vi "Contour Defect Inspection.vi"() -> ()   [LabVIEW 2016]
doc: "This example shows a contour analysis application. The contour of the rim of the can is extracted and a circle is fitted to those points. Then the contour is compared to the fitted circle to locate defects."
uses:
  <vilib>/vision/NI_Vision_Development_Module.lvlib
panel:
  out "Pass Status":bool
  in  "Max Distance":dbl=4.0 min=0.0 format="%.2f"
  out "Distance":dbl[](graph) caption="Distance of Contour from Fitted Circle"
  in  "Stop":bool
  out "Image":T1(plugin-control)
  in  "Delay (s.)":dbl(slide)=0.995260663507109 scale=0.0..3.0
  # "Overview: Demonstrates how to use the IMAQ Fit Contour function to compare the extracted contour against an expected shape contour and IMAQ Compute Contour Distance calculates the distance of the contour points from the expected shape.\nRequirements: Vision Development Software.\nInstructions:\n1. Run the VI.\n2. Adjust the Max Distance to change the distance tolerance. The locations that are greater than this maximum distance are overlaid in red on the image."
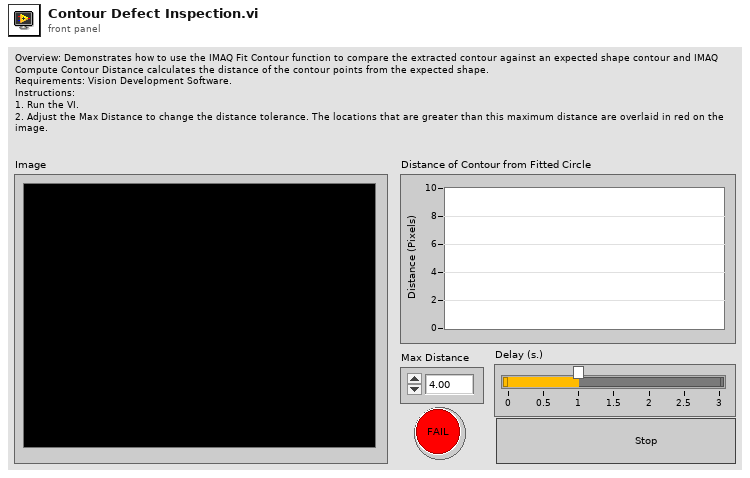
[diagram p1: front panel]
types:
  T1 = typedef "IMAQ Image.ctl" = refnum<image>
  T2 = typedef "IMAQ Circle" = cluster{"Center X":i32, "Center Y":i32, "Inner Radius":i32, "Outer Radius":i32, "Start Angle":dbl, "End Angle":dbl}
  T3 = typedef "ROI Descriptor" = cluster{"Global Rectangle":i32[], "Contours":cluster{"ID":enum32{"External", "Internal"}, "Type":u32, "Coordinates":i32[]}[]}
  T4 = cluster{"Overlay?":bool, "Color":u32, "Width":u32, "Maintain Width?":bool}
  T5 = enum16{"Closest To Search Start", "Maximum Length", "Strongest Mean Gradient Change"}
  T6 = enum16{"Rect Left To Right", "Rect Right To Left", "Rect Top To Bottom", "Rect Bottom To Top", "Annulus Inner To Outer", "Annulus Outer To Inner", "Annulus Start Angle To End Angle", "Annulus End Angle To Start Angle"}
  T7 = cluster{"Target Point":cluster{"X":dbl, "Y":dbl}, "Template Point":cluster{"X":dbl, "Y":dbl}, "Distance":dbl}[]
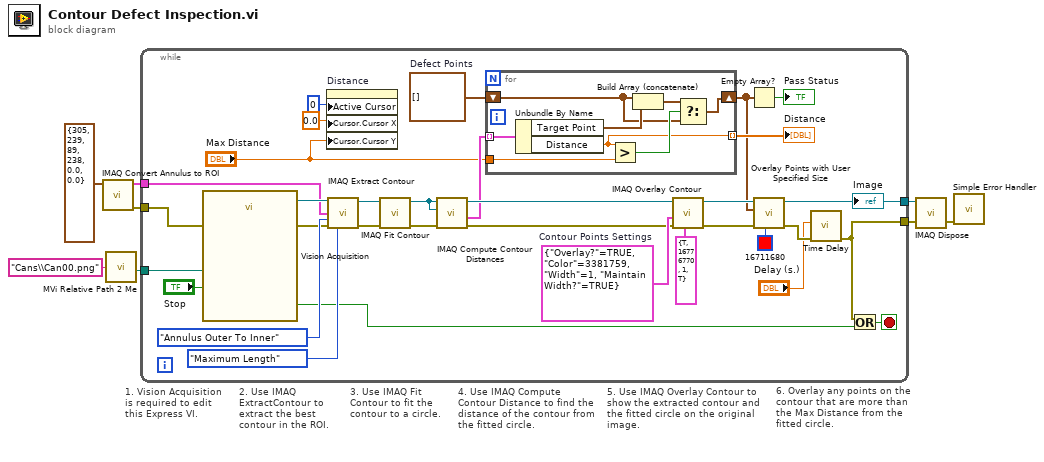
[diagram p0: block diagram]
diagram:
  # "1. Vision Acquisition is required to edit this Express VI."
  # "6. Overlay any points on the contour that are more than the Max Distance from the fitted circle."
  # "4. Use IMAQ Compute Contour Distance to find the distance of the contour from the fitted circle."
  # "3. Use IMAQ Fit Contour to fit the contour to a circle."
  # "5. Use IMAQ Overlay Contour to show the extracted contour and the fitted circle on the original image."
  # "2. Use IMAQ ExtractContour to extract the best contour in the ROI."
  n1 = call "IMAQ Convert Annulus to ROI"("Annulus"=T2 {"Center X"=305, "Center Y"=239, "Inner Radius"=89, "Outer Radius"=238, "Start Angle"=0.0, "End Angle"=0.0}) -> ("error out"=w3:errorcluster, "ROI Descriptor"=w6:T3)  [unwired: 8 in]
  n2 = call "MVi Relative Path 2 Me.vi"("Relative Path"="Cans\\Can00.png" ("name or relative path")) -> ("Appended Dir"=w2:path)  [unwired: 5 in, 1 out]
  n3 = while {
    tunnel: [w25] -> w8
    tunnel: w2 -> [w22]
    tunnel: w6 -> [w21]
    tunnel: [w11] -> w5
    tunnel: w3 -> [w12]
    stop <- w10 stop-if-true
    w28 = cluster{"X":dbl, "Y":dbl}[] []  # Defect Points
    w38 = T4 {"Overlay?"=TRUE, "Color"=3381759, "Width"=1, "Maintain Width?"=TRUE}  # Contour Points Settings
    n4 = call "Vision Acquisition"("Image Path"=w22, "Stop (F)"="Stop", "error in"=w12) -> ("Image Out"=w24:T1, "Stopped"=w9:bool, "error out"=w23:errorcluster)  [unwired: 22 in]
    n5 = property on="Distance" class="WFGraph (strict)"("Active Cursor"=u32 0, "Cursor.Cursor X"=0.0 ("Cursor.Cursor Position:Cursor X"), "Cursor.Cursor Y"="Max Distance") -> ()  [unwired: 2 in, 2 out]
    n6 = call "IMAQ Extract Contour"("Source Image"=w24, "ROI Descriptor"=w21, "Search Direction"=T6."Annulus Outer To Inner", "error in (no error)"=w23, "Contour Selection"=T5."Maximum Length") -> ("Source Image Out"=w34:T1, "error out"=w33:errorcluster)  [unwired: 3 in, 6 out]
    n7 = call-poly "IMAQ Fit Contour"("error in (no error)"=w33, "Contour Image"=w34) -> ("error out"=w39:errorcluster, "Contour Image Out"=w30:T1)  [unwired: 2 in, 6 out]
    n8 = call "IMAQ Compute Contour Distances"("error in (no error)"=w39, "Template Contour Image"=w30, "Target Contour Image"=w30) -> ("error out"=w35:errorcluster, "Distances"=w29:T7, "Target Contour Image Out (dup)"=w36:T1)  [unwired: 2 in, 4 out]
    n9 = for {
      tunnel: w29 -> [w49] mode=indexing
      shift-right: [w44] -> w19
      shift-left: w28 -> [w45]
      tunnel: [w43] -> w20 mode=indexing
      tunnel: "Max Distance" -> [w42]
      n10 = Unbundle By Name(w49) -> ("Target Point"=w48:cluster{"X":dbl, "Y":dbl}, "Distance"=w43:dbl)
      n11 = Greater?(x=w43, y=w42) -> (0:w47:bool)
      n12 = Build Array (concatenate)(w45, w48) -> (w46:cluster{"X":dbl, "Y":dbl}[])
      n13 = Select(t=w46, s=w47, f=w45) -> (s? t:f=w44:cluster{"X":dbl, "Y":dbl}[])
    }
    "Distance" <- w20
    n14 = call "IMAQ Overlay Contour"("Contour Equation Settings"=T4 {"Overlay?"=TRUE, "Color"=16776770, "Width"=1, "Maintain Width?"=TRUE}, "error in (no error)"=w35, "Contour Points Settings"=w38, "Image"=w36) -> ("error out"=w13:errorcluster, "Image Out"=w27:T1)  [unwired: 2 in, 4 out]
    n15 = Empty Array?(array=w19) -> (empty?=→"Pass Status":bool)
    n16 = call "Overlay Points with User Specified Size.vi"("Color"=u32 16711680, "error in"=w13, "Points"=w19, "Image In"=w27) -> ("error out"=w15:errorcluster, "Image Out"=w25:T1)  [unwired: 6 in]
    "Image" <- w25
    n17 = call "Time Delay"("error in (no error)"=w15, "Delay Time (s)"="Delay (s.)") -> ("error out"=w11:errorcluster)  [unwired: 9 in]
    n18 = Or(x=w11, y=w9) -> (x .or. y?=w10:bool)
  }
  n19 = call "IMAQ Dispose"("Image"=w8, "error in (no error)"=w5) -> ("error out"=w4:errorcluster)  [unwired: 1 in, 3 out]
  n20 = call <vilib>:"Simple Error Handler.vi"("error in (no error)"=w4) -> ()  [unwired: 4 in, 5 out]
